vi "passTestAllResults.vi"() -> ()   [LabVIEW 2017]
uses:
  passTestStates.ctl
panel:
  in  "Result":T1
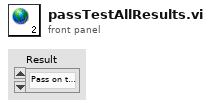
[diagram p1: front panel]
types:
  T1 = typedef "passTestStates.ctl" = enum16{"Pass on the way", "Ball stops", "Pass intercepted", "Ball out of the field", "Ball missed robot", "Need more force to pass", "Too much force", "Correct pass", "Keep ball possesion", "Robot kicked the ball", "Waiting Kick", "Invalid: same robot", "Invalid: kicker ID 999", "Invalid: Receiver ID 999", "Invalid"}
diagram:
